vi "Translator.CleanupControls.vi"(7 "VI name":string, 8 "error in":errorcluster, 10 "Controls":T1[](array[typedef])) -> (0 "error out":errorcluster)   [LabVIEW 2016]
uses:
  Translator.ControlData.ctl
  Translator.ControlTypes.ctl
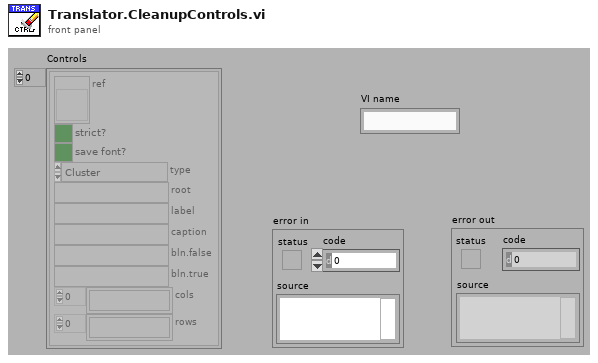
[diagram p1: front panel]
types:
  T1 = typedef "Translator.ControlData.ctl" = cluster{"ref":refnum<vi>, "strict?":bool, "save font?":bool, "type":T2, "root":string, "label":string, "caption":string, "bln.false":string, "bln.true":string, "cols":string[], "rows":string[]}
  T2 = typedef "Translator.ControlTypes.ctl" = enum16{"Cluster", "Array", "Boolean", "Ring", "String", "Tab", "Listbox", "Multicolumn listbox", "Table", "Tree", "Other"}
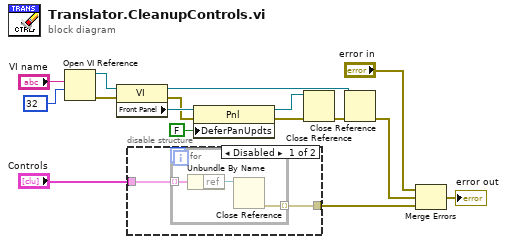
[diagram p0: block diagram]
diagram:
  n1 = Open VI Reference(vi path="VI name", options=32) -> (vi reference=w5:refnum<vi>, error out=w12:errorcluster)  [unwired: 1 in, 3 out]
  n2 = property class="VI"(reference=w5, error in=w12) -> (reference out=w6:refnum<vi>, error out=w11:errorcluster, "Front Panel"=w13:refnum<vi>)
  n3 = disable-structure shown="Disabled" {
    disable-tunnel: "Controls" -> [w18 _]
    disable-tunnel: [w17 _] -> w15
    frame Disabled {
      n4 = for {
        tunnel: w18 -> [w21] mode=indexing
        tunnel: [w19] -> w17 mode=indexing
        n5 = Unbundle By Name(w21) -> ("ref"=w20:refnum<vi>)
        n6 = Close Reference(reference=w20) -> (error out=w19:errorcluster)  [unwired: 1 in]
      }
    }
    frame Enabled {
    }
  }
  n7 = property class="Pnl"(reference=w13, error in=w11, "DeferPanUpdts"=FALSE ("Defer Panel Updates")) -> (reference out=w7:refnum<vi>, error out=w8:errorcluster)
  n8 = Close Reference(reference=w7, error in (no error)=w8) -> (error out=w10:errorcluster)
  n9 = Close Reference(reference=w6, error in (no error)=w10) -> (error out=w4:errorcluster)
  n10 = Merge Errors("error in", w4, w15) -> (→"error out":errorcluster)
